vi "PH_Sixpack.destructor.vi"(0 "i ref in":refnum<vi>, 5 "error in":errorcluster) -> (19 "error out":errorcluster)   [LabVIEW 2014, in "PH_Sixpack.lvlib"]
doc: "This is the destructor of a class.\n\nLicense Agreement for this software:\n\nCopyright (C)\nGesellschaft für Schwerionenforschung, GSI\nPlanckstr. 1\n64291 Darmstadt\nGermany\n\nContact: D.Beck@gsi.de \n\nThis program is free software; you can redistribute it and/or modify it under the terms of the \nGNU General Public License as published by the Free Software Foundation; either version 2 of \nthe license, or (at your option) any later version.\n\nThis program is distributed in the hope that it will be useful, but WITHOUT ANY WARRANTY; \nwithout even the implied warranty of MERCHANTABILITY or FITNESS FOR A PARTICULAR PURPOSE. See the GNU General License for more details (http://www.gnu.org).\n\nGesellschaft für Schwerionenforschung, GSI\nPlanckstr. 1, 64291 Darmstadt, Germany\nFor all questions and ideas contact: M.Richter@gsi.de, H.Brand@gsi.de or D.Beck@gsi.de.\nLast update: 16-JUN-2004"
uses:
  PH_Sixpack.lvlib
  PH_Sixpack.Status.ctl
  PH_Stepmotor_BaseClass/PH_Stepmotor_BaseClass.lvlib
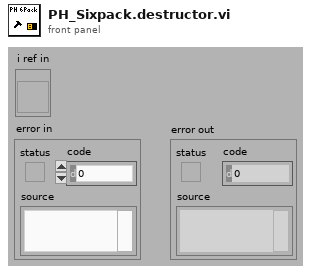
[diagram p1: front panel]
types:
  T1 = typedef "PH_Sixpack.lvlib/PH_Sixpack.Status.ctl" = enum32{"None", "Init", "Configure", "configured", "Close", "closed"}
  T2 = enum16{"SetAttribute", "GetAttribute", "CreateAttribute", "DestroyAttribute", "DestroyAllAtributes"}
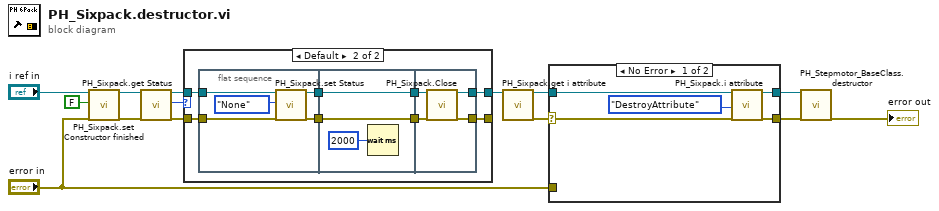
[diagram p0: block diagram]
diagram:
  n1 = call "PH_Sixpack.set Constructor finished.vi"("VI in"="i ref in", "Constructor finished?"=FALSE, "error in (no error)"="error in") -> ("VI out"=w7:refnum<vi>, "error out"=w10:errorcluster)  [unwired: 15 in]
  n2 = call "PH_Sixpack.get Status.vi"("VI in"=w7, "error in (no error)"=w10) -> ("VI out"=w12:refnum<vi>, "Status"=w11:T1, "error out"=w13:errorcluster)  [unwired: 14 in, 1 out]
  n3 = case shown="Default" w11 {
    tunnel: w13 -> [w15 w20]
    tunnel: [w15 w19] -> _
    tunnel: w12 -> [w16 w18]
    tunnel: [w16 w17] -> w4
    frame "None", "Init", "closed" {
    }
    frame Default {
      n4 = flat-sequence {
        tunnel: w20 -> [w29]
        tunnel: w18 -> [w27]
        tunnel: [w28] -> w24
        tunnel: [w26] -> w23
        tunnel: w24 -> [w32]
        tunnel: w23 -> [w31]
        tunnel: [w32] -> w22
        tunnel: [w31] -> w21
        tunnel: [w35] -> w17
        tunnel: [w33] -> w19
        tunnel: w22 -> [w34]
        tunnel: w21 -> [w36]
        frame #0 {
          n5 = call "PH_Sixpack.set Status.vi"("VI in"=w27, "Status"=PH_Sixpack.Status."None", "error in (no error)"=w29) -> ("VI out"=w26:refnum<vi>, "error out"=w28:errorcluster)  [unwired: 15 in]
        }
        frame #1 {
          n6 = Wait (ms)(milliseconds to wait=u32 2000) -> ()  [unwired: 1 out]
        }
        frame #2 {
          n7 = call "PH_Sixpack.Close.vi"("i ref in"=w36, "error in (no error)"=w34) -> ("i ref out"=w35:refnum<vi>, "error out"=w33:errorcluster)  [unwired: 16 in]
        }
      }
    }
  }
  n8 = call "PH_Sixpack.get i attribute.vi"("i ref in"=w4) -> ("i ref out"=w5:refnum<vi>, "error out"=w3:errorcluster)  [unwired: 16 in, 1 out]
  n9 = case shown="No Error" w3 {
    selector: w3 -> [w37 _]
    tunnel: [w40 w42] -> w14
    tunnel: [w39 w43] -> w6
    tunnel: w5 -> [w38 w43]
    tunnel: "error in" -> [_ w42]
    frame No Error {
      n10 = call "PH_Sixpack.i attribute.vi"("VI Refnum"=w38, "Action"=T2."DestroyAttribute", "error in (no error)"=w37) -> ("VI Refnum out"=w39:refnum<vi>, "error out"=w40:errorcluster)  [unwired: 14 in, 1 out]
    }
    frame Error {
    }
  }
  n11 = call "PH_Stepmotor_BaseClass.destructor.vi"("i ref in"=w6, "error in"=w14) -> ("error out"=→"error out":errorcluster)  [unwired: 17 in]
